vi "Plot J profile.vi"(5 "p0":dbl, 6 "Steps":i32, 7 "flux":dbl, 8 "error in (no error)":errorcluster, 11 "path in":path) -> (0 "error out":errorcluster, 2 "plot":cluster{cluster{dbl, "return type":dbl}[]}, 3 "path out":path)   [LabVIEW 2023]
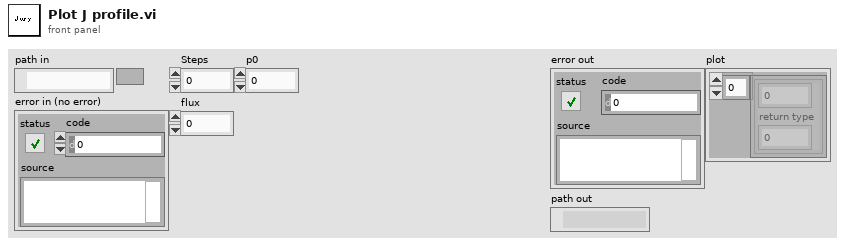
[diagram p1: front panel]
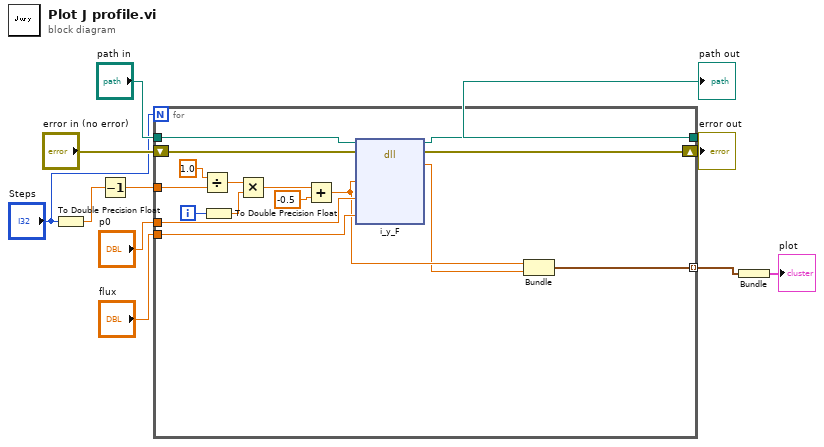
[diagram p0: block diagram]
diagram:
  n1 = To Double Precision Float(number="Steps") -> (double precision float=w4:dbl)
  n2 = Decrement(x=w4) -> (x-1=w3:dbl)
  n3 = for {
    N: "Steps" -> [_]
    shift-right: [w25] -> w9
    shift-left: "error in (no error)" -> [w26]
    tunnel: "path in" -> [w27]
    tunnel: [w24] -> w8
    tunnel: "flux" -> [w23]
    tunnel: "p0" -> [w22]
    tunnel: w3 -> [w20]
    tunnel: [w12] -> w2 mode=indexing
    i -> [w18]
    n4 = Divide(x=1.0, y=w20) -> (x/y=w19:dbl)
    n5 = To Double Precision Float(number=w18) -> (double precision float=w17:dbl)
    n6 = Multiply(x=w19, y=w17) -> (x*y=w16:dbl)
    n7 = Add(x=w16, y=-0.5) -> (x+y=w14:dbl)
    n8 = dll-call lib="C:/Users/yg/Box/Guang Yue uiuc research box folder/computation/S-TI-S jj simulation c/Release/ygDLL.dll" fn="i_y_F"(path in=w27, error in=w26, "y"=w14, "p0"=w22, "flux"=w23) -> (path out=w24:path, error out=w25:errorcluster, "return type"=w13:dbl)  [unwired: 4 in]
    n9 = Bundle(w14, "return type"=w13) -> (w12:cluster{dbl, "return type":dbl})  [unwired: 1 in]
  }
  "error out" <- w9
  "path out" <- w8
  n10 = Bundle(w2) -> (→"plot":cluster{cluster{dbl, "return type":dbl}[]})  [unwired: 1 in]
